vi "Get Plugin Pointers.vi"(8 "error in (no error)":errorcluster, 10 "plugin index":i32, 11 "Framework Status in":refnum<class "Framework Status.lvclass">) -> (0 "error out":errorcluster, 1 "group status pointers":refnum<class "Status Pointer.lvclass">[](array[class]), 2 "plugin status pointer":refnum<class "Status Pointer.lvclass">, 3 "Framework Status out":refnum<class "Framework Status.lvclass">)   [LabVIEW 2020, in "DSF Core.lvlib" / "Framework Status.lvclass"]
uses:
  Framework Status.lvclass
  Status/Status Pointer.lvclass
  C:/Program Files (x86)/National Instruments/LabVIEW 2020/vi.lib/NI/Memory Manager/Classes/Pointer/Pointer.lvclass
  Framework Status.lvclass/Framework Status.ctl
  <vilib>/NI/Memory Manager/Classes/Pointer/Pointer.lvclass/Pointer.ctl
  <vilib>/NI/Memory Manager/Classes/Pointer/Subset.vi
  Status/Status Size.vi
  <vilib>/NI/Memory Manager/Classes/Pointer/Get Address.vi
  <vilib>/NI/Memory Manager/Classes/Pointer/Encapsulate.vi
  <vilib>/NI/Memory Manager/Classes/Pointer/Check Null Pointer.vi
  <vilib>/NI/Memory Manager/Classes/Pointer/Check Length.vi
  <vilib>/NI/Memory Manager/Classes/Pointer/Set Size.vi
  <vilib>/NI/Memory Manager/Classes/Pointer/Set Address.vi
  <vilib>/NI/Memory Manager/Classes/Pointer/Set Internal.vi
  <vilib>/NI/Memory Manager/Classes/Pointer/Errors.vi
  <vilib>/NI/Memory Manager/Classes/Pointer/Null Pointer.vi
  <vilib>/NI/Memory Manager/Classes/Pointer/Is Null.vi
  <vilib>/NI/Memory Manager/Classes/Pointer/Get Size.vi
  <vilib>/NI/Memory Manager/Classes/Pointer/Check Bounds (Pointer).vi
  <vilib>/NI/Memory Manager/Classes/Pointer/Create Error.vi
  <vilib>/NI/Memory Manager/Classes/Pointer/Out of Bounds.vi
  <vilib>/NI/Memory Manager/VIs/New Error Cluster.vi
  <vilib>/NI/Memory Manager/VIs/New Error Cluster (512B).vi
  <vilib>/NI/Memory Manager/VIs/Set Error Status.vi
  <vilib>/NI/Memory Manager/VIs/Set Error Code.vi
  <vilib>/NI/Memory Manager/VIs/Set Error Source.vi
  <vilib>/NI/Memory Manager/Constants/Constants.vi
  <vilib>/NI/Memory Manager/Constants/Library Name.vi
  <vilib>/NI/Memory Manager/Classes/Pointer/Pointer Error Info.vi
  <vilib>/NI/Memory Manager/VIs/Write String to Source.vi
  <vilib>/NI/Memory Manager/Constants/Pointer Class Name.vi
  <vilib>/NI/Memory Manager/Classes/Pointer/Write Pointer Size to Error.vi
  <vilib>/NI/Memory Manager/VIs/Write Numeric to Source.vi
  <vilib>/NI/Memory Manager/VIs/Write Numeric Scalar to Source (Base10 U64).vi
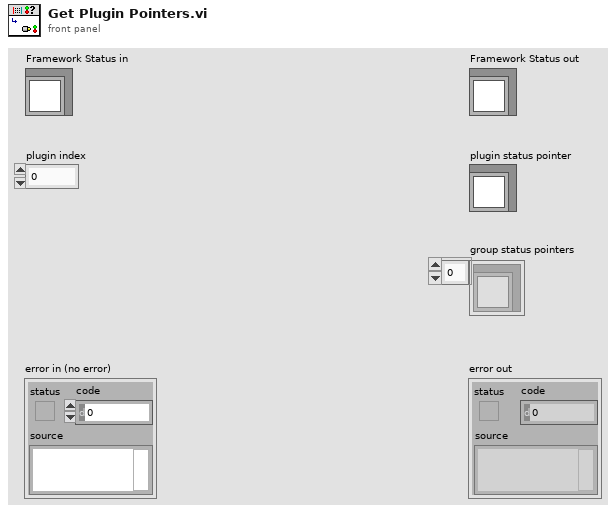
[diagram p1: front panel]
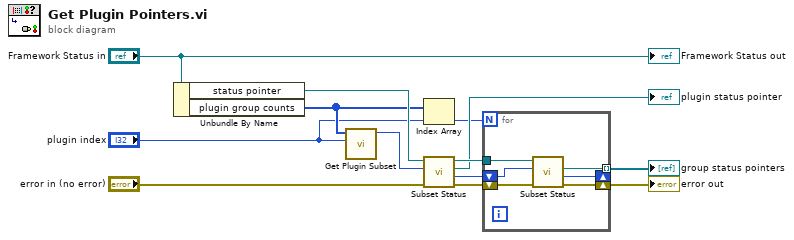
[diagram p0: block diagram]
diagram:
  n1 = Unbundle By Name("Framework Status in") -> ("status pointer"=w10:refnum<class "Status Pointer.lvclass">, "plugin group counts"=w9:u8[])
  n2 = call "Get Plugin Subset.vi"("plugin index"="plugin index", "plugin group counts"=w9) -> ("index"=w12:i32)  [unwired: 8 in, 1 out]
  n3 = Index Array(array=w9, index="plugin index") -> (element=w2:u8)
  n4 = call "Subset Status.vi"("error in (no error)"="error in (no error)", "index"=w12, "status pointer in"=w10) -> ("error out"=w7:errorcluster, "index + count"=w6:u64, "subset status pointer"=→"plugin status pointer":refnum<class "Status Pointer.lvclass">, "status pointer out"=w5:refnum<class "Status Pointer.lvclass">)  [unwired: 5 in]
  n5 = for {
    N: w2 -> [_]
    shift-right: [w18] -> w1
    shift-left: w7 -> [w19]
    shift-right: [w16] -> _
    shift-left: w6 -> [w17]
    tunnel: w5 -> [w15]
    tunnel: [w14] -> w3 mode=indexing
    n6 = call "Subset Status.vi"("error in (no error)"=w19, "index"=w17, "status pointer in"=w15) -> ("error out"=w18:errorcluster, "index + count"=w16:u64, "subset status pointer"=w14:refnum<class "Status Pointer.lvclass">)  [unwired: 5 in, 1 out]
  }
  "error out" <- w1
  "group status pointers" <- w3
  "Framework Status out" <- "Framework Status in"
